vi "FindXYandT.vi"(11 "path":path=path "/Users/milandahal/Downloads/ED-R Videos/Ramp 480p/ramp-480p - 30fps ") -> (2 "Image":picture, 3 "Array":dbl[][](array[numeric]))   [LabVIEW 2021]
uses:
  <userlib>/ImageProcessing/IdentifyBlob_Circle_Cluster.vi
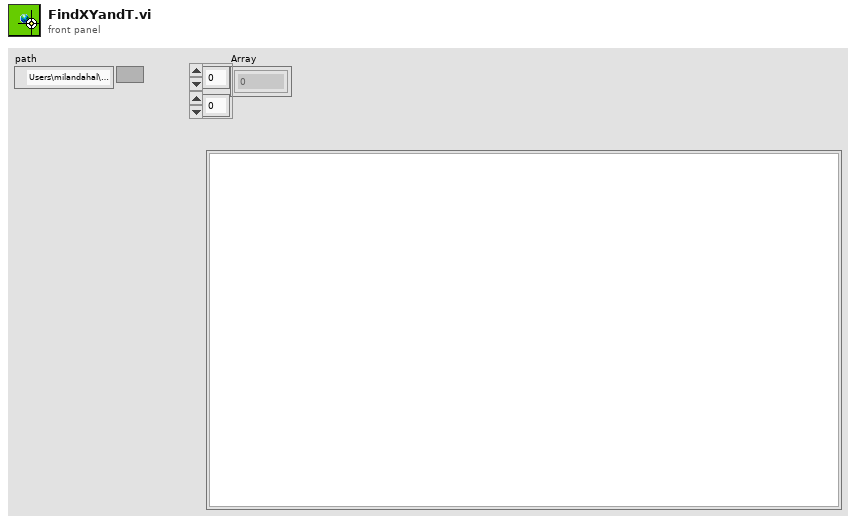
[diagram p1: front panel]
types:
  T1 = typedef "QT_Image.ctl" = cluster{"Width":i32, "Height":i32, "Depth":i32, "data":u8[], "Compressed data":u8[], "Color table":u32[], "Duration":i32, "Options":i32, "Timestamp":i32, "ID":i32, "Reserved":i32, "Dialogs":u32}
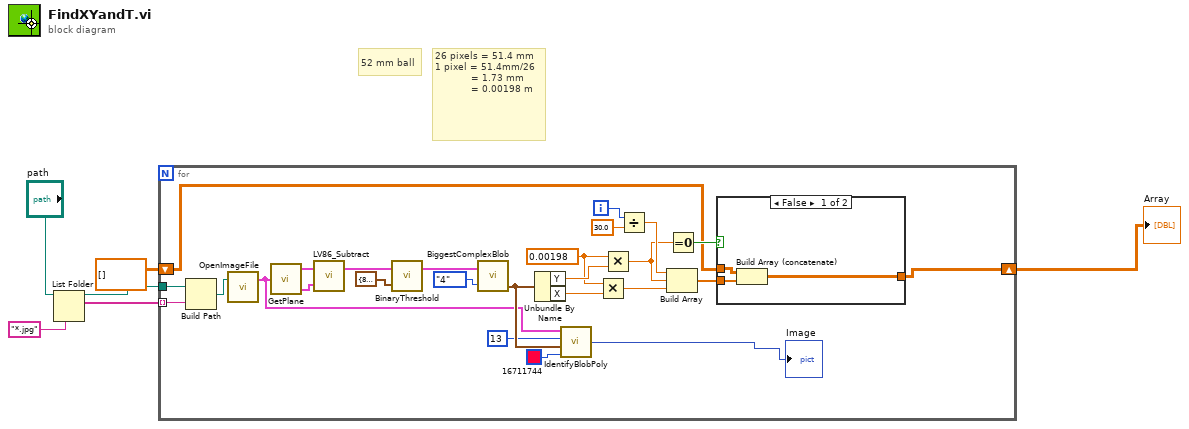
[diagram p0: block diagram]
diagram:
  # "26 pixels = 51.4 mm\n1 pixel = 51.4mm/26\n            = 1.73 mm\n            = 0.00198 m"
  # "52 mm ball"
  n1 = List Folder(path="path", pattern="*.jpg" ("string")) -> (path out=w4:path, filenames=w2:string[])  [unwired: 2 in, 2 out]
  n2 = for {
    tunnel: w2 -> [w31] mode=indexing
    tunnel: w4 -> [w32]
    shift-right: [w22] -> w6
    shift-left: dbl[][] [] -> [w24]
    i -> [w20]
    w12 = 0.00198 ("x")
    n3 = Build Path(base path=w32, name or relative path=w31) -> (appended path=w30:path)
    n4 = call <userlib>:"OpenImageFile.vi"("selected path"=w30) -> ("Image Out"=w18:T1)  [unwired: 2 in]
    n5 = call <userlib>:"GetPlane.vi"("Image In"=w18) -> ("Blue Plane Out"=w17:T1, "Red Plane Out"=w16:T1)  [unwired: 1 out]
    n6 = call <userlib>:"LV86_Subtract.vi"("Image 2"=w17, "Image"=w16) -> ("Image Out"=w15:T1)  [unwired: 1 in]
    n7 = call <userlib>:"BinaryThreshold.vi"("threshold"=cluster{u8, u8} {82, 120} ("Red Threshold"), "Image In"=w15) -> ("Image Out"=w14:T1)  [unwired: 1 in]
    n8 = call <userlib>:"BiggestComplexBlob.vi"("Connectivity"=enum16{"4", "8"}."4", "Image in"=w14) -> ("Centroid"=w29:cluster{"X":dbl, "Y":dbl})  [unwired: 2 out]
    n9 = Unbundle By Name(w29) -> ("Y"=w26:dbl, "X"=w11:dbl)
    n10 = call-poly <userlib>:"IdentifyBlobPoly.vi"("color"=u32 16711744, "Centroid"=w29, "Dimension"=13, "Image in"=w18) -> ("picture"=→"Image":picture)
    n11 = Multiply(x=w12, y=w11) -> (x*y=w10:dbl)
    n12 = Multiply(x=w12, y=w26) -> (x*y=w8:dbl)
    n13 = Divide(x=w20, y=30.0 ("x")) -> (x/y=w9:dbl)
    n14 = Build Array(w9, w8, w10) -> (w23:dbl[])
    n15 = Equal To 0?(x=w8) -> (x = 0?=w25:bool)
    n16 = case shown="False" w25 {
      tunnel: w24 -> [w35 w36]
      tunnel: w23 -> [w34 _]
      tunnel: [w33 w36] -> w22
      frame False {
        n17 = Build Array (concatenate)(w35, w34) -> (w33:dbl[][])
      }
      frame True {
        # "to remove all 0 centroids"
      }
    }
  }
  "Array" <- w6
